vi "LockInResistanceMeasurement.vi"(7 "Stanford Error In":errorcluster, 8 "Temperature":dbl, 9 "Keithley Current":dbl, 10 "Stanford ID":refnum<visa-resource-name>) -> (0 "error out":errorcluster, 1 "Stanford ID":refnum<visa-resource-name>, 2 "output cluster":T1, 3 "Device Resistance":dbl)   [LabVIEW 2013]
doc: "This example shows how to configure the instrument to read all the parameters available."
uses:
  StanfordVoltage.vi
  temp-global.vi
  field-global.vi
  I-AC-global.vi
  resistance-global.vi
  IntegrationTime-global.vi
  <instrlib>/Stanford Research 830/Public/Data/Read (All Parameters).vi
  <instrlib>/Stanford Research 830/Stanford Research 830.lvlib
panel:
  # "(c) 2006 National Instruments.  ALL RIGHTS RESERVED."
  # "READOUT"
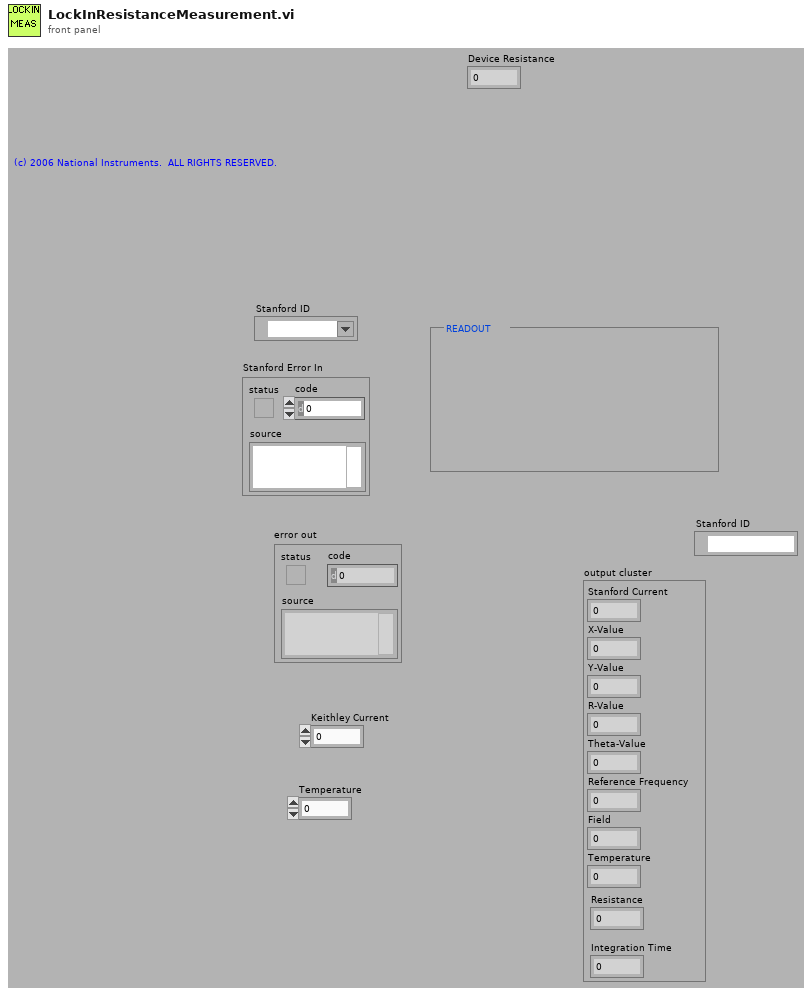
[diagram p1: front panel]
types:
  T1 = cluster{"Stanford Current":dbl, "X-Value":dbl, "Y-Value":dbl, "R-Value":dbl, "Theta-Value":dbl, "Reference Frequency":dbl, "Field":dbl, "Temperature":dbl, "Resistance":dbl, "Integration Time":dbl}
  T2 = cluster{"X-Value":dbl, "Y-Value":dbl, "R-Value":dbl, "Theta-Value":dbl, "Aux In 1 Value":dbl, "Aux In 2 Value":dbl, "Aux In 3 Value":dbl, "Aux In 4 Value":dbl, "Reference Frequency":dbl, "Channel 1 Display":dbl, "Channel 2 Display":dbl}
  T3 = cluster{dbl, "X-Value":dbl, "Y-Value":dbl, "R-Value":dbl, "Theta-Value":dbl, "Reference Frequency":dbl, "Field":dbl, "Temperature":dbl, dbl, dbl}
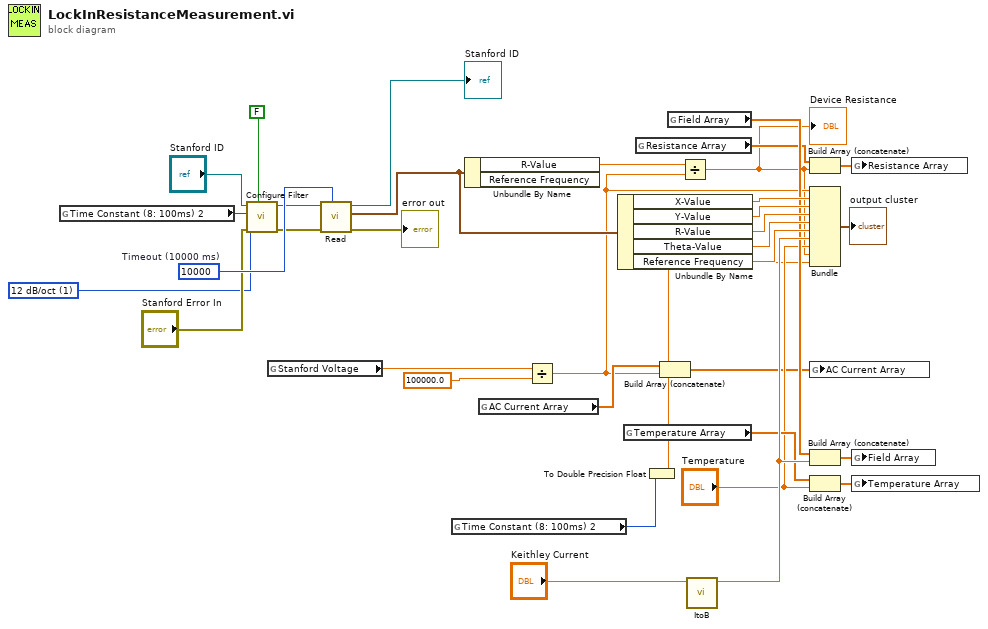
[diagram p0: block diagram]
diagram:
  w2 = u16 1 items=["6 dB/oct", "12 dB/oct", "18 db/oct", "24 dB/oct"] ("Low Pass Filter Slope (1: 12dB/oct)")
  w35 = u32 10000  # Timeout (10000 ms)
  n1 = global read "IntegrationTime-global.vi" "Time Constant (8: 100ms) 2"() -> (w6:u16)
  n2 = call <instrlib>:"Configure Filter.vi"("Enable Sync Filter (F: Disable)"=FALSE, "error in (no error)"="Stanford Error In", "Low Pass Filter Slope (1: 12dB/oct)"=w2, "Time Constant (8: 100ms)"=w6, "VISA resource name"="Stanford ID") -> ("error out"=w9:errorcluster, "VISA resource name out"=w10:refnum<visa-resource-name>)  [unwired: 5 in]
  n3 = global read "StanfordVoltage.vi" "Stanford Voltage"() -> (w31:dbl)
  n4 = call-poly <instrlib>:"Read.vi"("Timeout (10000 ms)"=w35, "error in (no error)"=w9, "VISA resource name"=w10) -> ("error out"=→"error out":errorcluster, "Parameter Values"=w29:T2, "VISA resource name out"=→"Stanford ID":refnum<visa-resource-name>)  [unwired: 6 in]
  n5 = global read "IntegrationTime-global.vi" "Time Constant (8: 100ms) 2"() -> (w5:u16)
  n6 = Unbundle By Name(w29) -> ("R-Value"=w30:dbl)  [unwired: 1 out]
  n7 = global read "I-AC-global.vi" "AC Current Array"() -> (w16:dbl[])
  n8 = Divide(x=w31, y=100000.0) -> (x/y=w15:dbl)
  n9 = Unbundle By Name(w29) -> ("X-Value"=w28:dbl, "Y-Value"=w27:dbl, "R-Value"=w26:dbl, "Theta-Value"=w25:dbl, "Reference Frequency"=w24:dbl)
  n10 = global read "temp-global.vi" "Temperature Array"() -> (w19:dbl[])
  n11 = global read "resistance-global.vi" "Resistance Array"() -> (w13:dbl[])
  n12 = To Double Precision Float(number=w5) -> (double precision float=w4:dbl)
  n13 = Build Array (concatenate)(w16, w15) -> (w14:dbl[])
  n14 = global read "field-global.vi" "Field Array"() -> (w21:dbl[])
  n15 = Divide(x=w30, y=w15) -> (x/y=w12:dbl)
  "Device Resistance" <- w12
  n16 = call "ItoB.vi"("Current"="Keithley Current") -> ("Field"=w22:dbl)  [unwired: 10 in]
  n17 = Build Array (concatenate)(w13, w12) -> (w11:dbl[])
  n18 = Bundle(w15, "X-Value"=w28, "Y-Value"=w27, "R-Value"=w26, "Theta-Value"=w25, "Reference Frequency"=w24, "Field"=w22, "Temperature"="Temperature", w12, w4) -> (→"output cluster":T3)  [unwired: 1 in]
  n19 = global write "I-AC-global.vi" "AC Current Array"(w14) -> ()
  n20 = Build Array (concatenate)(w21, w22) -> (w20:dbl[])
  n21 = Build Array (concatenate)(w19, "Temperature") -> (w17:dbl[])
  n22 = global write "resistance-global.vi" "Resistance Array"(w11) -> ()
  n23 = global write "field-global.vi" "Field Array"(w20) -> ()
  n24 = global write "temp-global.vi" "Temperature Array"(w17) -> ()
